vi "GetMaximumStepNameLength.vi"(4 "error in (no error)":errorcluster, 7 "RuleConfiguration in":refnum<k7>) -> (0 "error out":errorcluster, 2 "Maximum Step Name Length":i32, 3 "RuleConfiguration out":refnum<k7>)   [LabVIEW 2011]
uses:
  StepNameLengthRuleConstants.vi
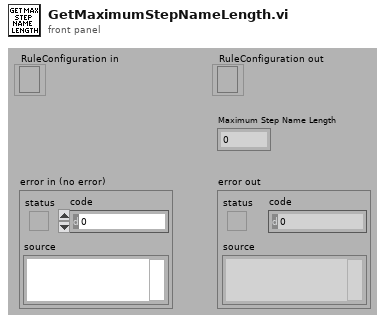
[diagram p1: front panel]
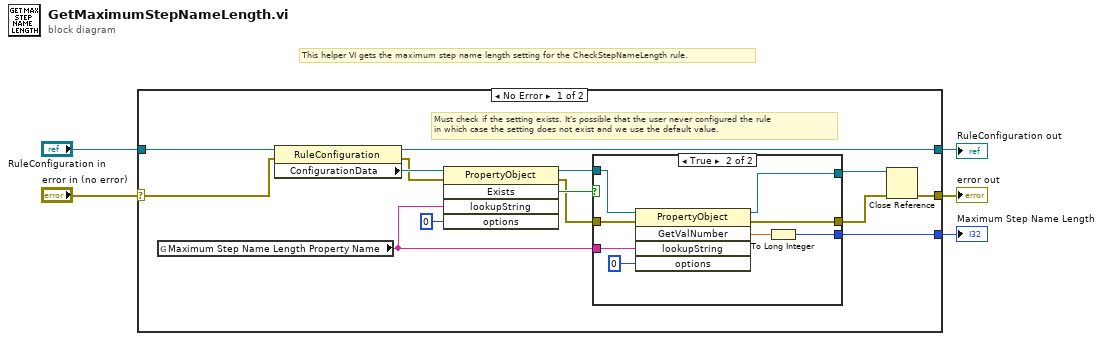
[diagram p0: block diagram]
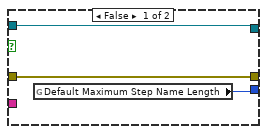
[diagram p2: hidden frame]
diagram:
  # "This helper VI gets the maximum step name length setting for the CheckStepNameLength rule."
  n1 = case shown="No Error" "error in (no error)" {
    selector: "error in (no error)" -> [w6 w31]
    tunnel: "RuleConfiguration in" -> [w19 w32]
    tunnel: [w14 _] -> w4
    tunnel: [w13 w32] -> w3
    tunnel: [w7 w31] -> w2
    frame No Error {
      # "Must check if the setting exists. It's possible that the user never configured the rule\nin which case the setting does not exist and we use the default value."
      n2 = global read "StepNameLengthRuleConstants.vi" "Maximum Step Name Length Property Name"() -> (w15:string)
      n3 = property class="RuleConfiguration"(reference=w19, error in=w6) -> (reference out=w13:refnum<k7>, error out=w12:errorcluster, "ConfigurationData"=w16:refnum<k7>)
      n4 = invoke class="PropertyObject" method="Exists"(reference=w16, error in=w12, "lookupString"=w15, "options"=0) -> (reference out=w10:refnum<k7>, error out=w11:errorcluster, "Exists"=w17:bool)  [unwired: 1 in, 2 out]
      n5 = case shown="True" w17 {
        tunnel: w10 -> [w20 w30]
        tunnel: w15 -> [_ w28]
        tunnel: [w22 w26] -> w14
        tunnel: w11 -> [w21 w25]
        tunnel: [w21 w24] -> w8
        tunnel: [w20 w23] -> w9
        frame False {
          n6 = global read "StepNameLengthRuleConstants.vi" "Default Maximum Step Name Length"() -> (w22:i32)
        }
        frame True {
          n7 = invoke class="PropertyObject" method="GetValNumber"(reference=w30, error in=w25, "lookupString"=w28, "options"=0) -> (reference out=w23:refnum<k7>, error out=w24:errorcluster, "GetValNumber"=w27:dbl)  [unwired: 1 in, 2 out]
          n8 = To Long Integer(number=w27) -> (32bit integer=w26:i32)
        }
      }
      n9 = Close Reference(reference=w9, error in (no error)=w8) -> (error out=w7:errorcluster)
    }
    frame Error {
    }
  }
  "Maximum Step Name Length" <- w4
  "RuleConfiguration out" <- w3
  "error out" <- w2
